vi "StartLegacy.vi"(7 "Alias Name":string, 8 "error in":errorcluster, 9 "Other Args":string, 10 "Port":i32, 11 "Micron Path":path) -> (0 "error out":errorcluster, 3 "Connection String":string)   [LabVIEW 2019]
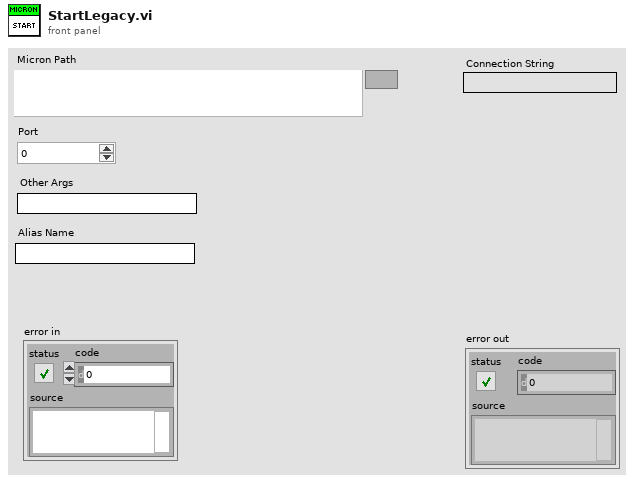
[diagram p1: front panel]
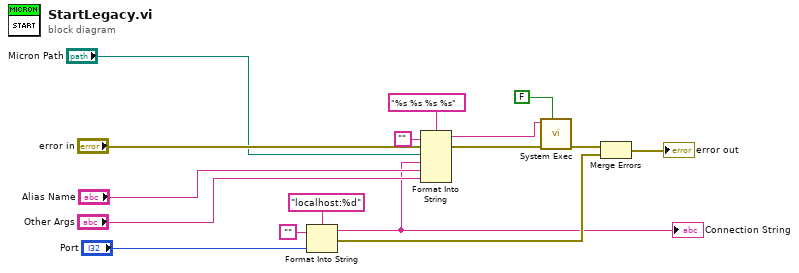
[diagram p0: block diagram]
diagram:
  n1 = Format Into String(format string="localhost:%d", initial string="", "Port") -> (resulting string=w2:string, error out=w3:errorcluster)  [unwired: 1 in]
  "Connection String" <- w2
  n2 = Format Into String(format string="%s %s %s %s", initial string="", error in="error in", "Micron Path", w2, "Alias Name", "Other Args") -> (resulting string=w12:string, error out=w15:errorcluster)
  n3 = call <vilib>:"System Exec.vi"("wait until completion? (T)"=FALSE, "error in (no error)"=w15, "command line"=w12) -> ("error out"=w8:errorcluster)  [unwired: 5 in, 3 out]
  n4 = Merge Errors(w8, w3) -> (→"error out":errorcluster)
